vi "deploy.vi"(8 "error in (no error)":errorcluster, 10 "build_spec":T1, 11 "lv-builder in":refnum<class "lv-builder.lvclass">) -> (0 "error out":errorcluster, 3 "lv-builder out":refnum<class "lv-builder.lvclass">)   [LabVIEW 2015, in "lv-builder.lvlib" / "lv-builder.lvclass"]
uses:
  lv-builder.lvclass
  lv-build/public/_controls/build_specification.ctl
  lv-build/public/_controls/build_type.ctl
  <vilib>/AppBuilder/AB_API_Simple/NI_App_Builder_API.lvlib
  lv-build/lv-build.lvlib
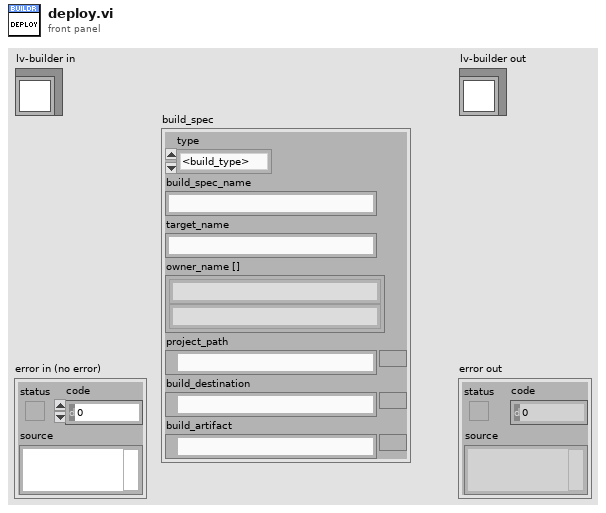
[diagram p1: front panel]
types:
  T1 = typedef "lv-build.lvlib/build_specification.ctl" = cluster{"type":T2, "build_spec_name":string, "target_name":string, "owner_name []":string[], "project_path":path, "build_destination":path, "build_artifact":path}
  T2 = typedef "lv-build.lvlib/build_type.ctl" = enum16{"<build_type>", "application_pc", "application_rt", "installer", "llb", "lvlibp", "zip", "fpga", "<null>"}
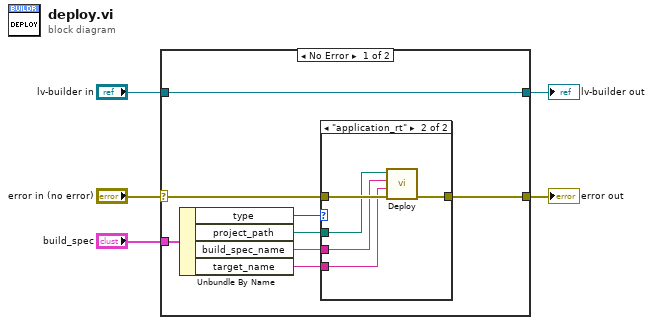
[diagram p0: block diagram]
diagram:
  n1 = case shown="No Error" "error in (no error)" {
    selector: "error in (no error)" -> [w12 w21]
    tunnel: [w11 w21] -> w2
    tunnel: "lv-builder in" -> [w7 w20]
    tunnel: "build_spec" -> [w13 _]
    tunnel: [w7 w20] -> w1
    frame No Error {
      n2 = Unbundle By Name(w13) -> ("type"=w6:T2, "project_path"=w10:path, "build_spec_name"=w9:string, "target_name"=w8:string)
      n3 = case shown="\"application_rt\"" w6 {
        tunnel: w12 -> [w14 w19]
        tunnel: [w14 w18] -> w11
        tunnel: w10 -> [_ w17]
        tunnel: w9 -> [_ w16]
        tunnel: w8 -> [_ w15]
        frame Default {
        }
        frame "application_rt" {
          n4 = call <vilib>:"Deploy.vi"("error in (no error)"=w19, "Name of target"=w15, "Name of build specification (if empty: deploy all)"=w16, "Path to project"=w17) -> ("error out"=w18:errorcluster)  [unwired: 7 in]
        }
      }
    }
    frame Error {
    }
  }
  "error out" <- w2
  "lv-builder out" <- w1
